vi "split by cursor pos.vi"(8 "error in":errorcluster, 11 "input":string) -> (0 "error out":errorcluster, 1 "Last cursor pos":cluster{i32, i32}, 2 "Sections":string[](array[string]), 3 "data":cluster{"Y":i32, "X":i32, "Text":string}[](array[cluster]))   [LabVIEW 2018]
uses:
  CAEN globals.vi
  <vilib>/regexp/Match Regular Expression.xnode
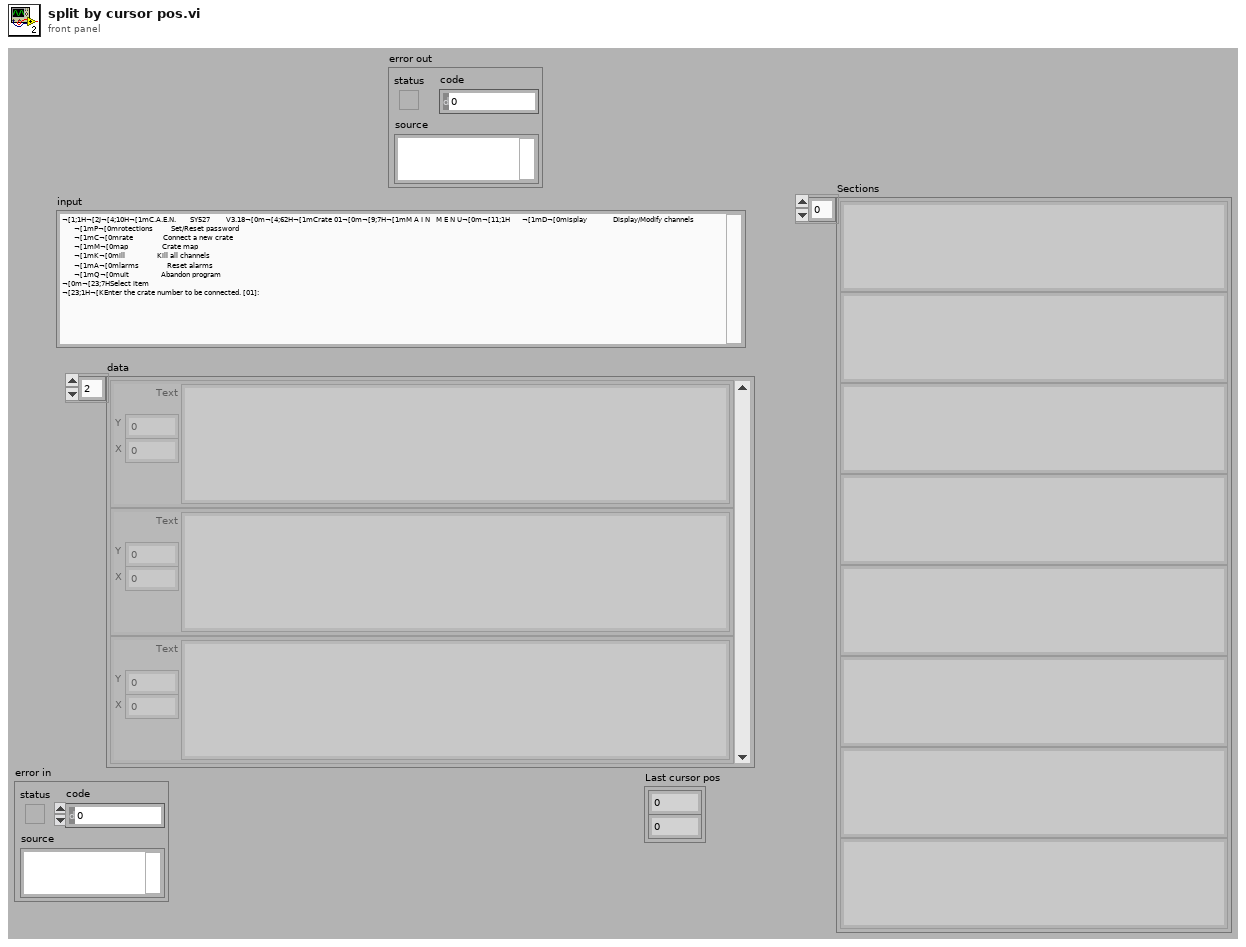
[diagram p1: front panel]
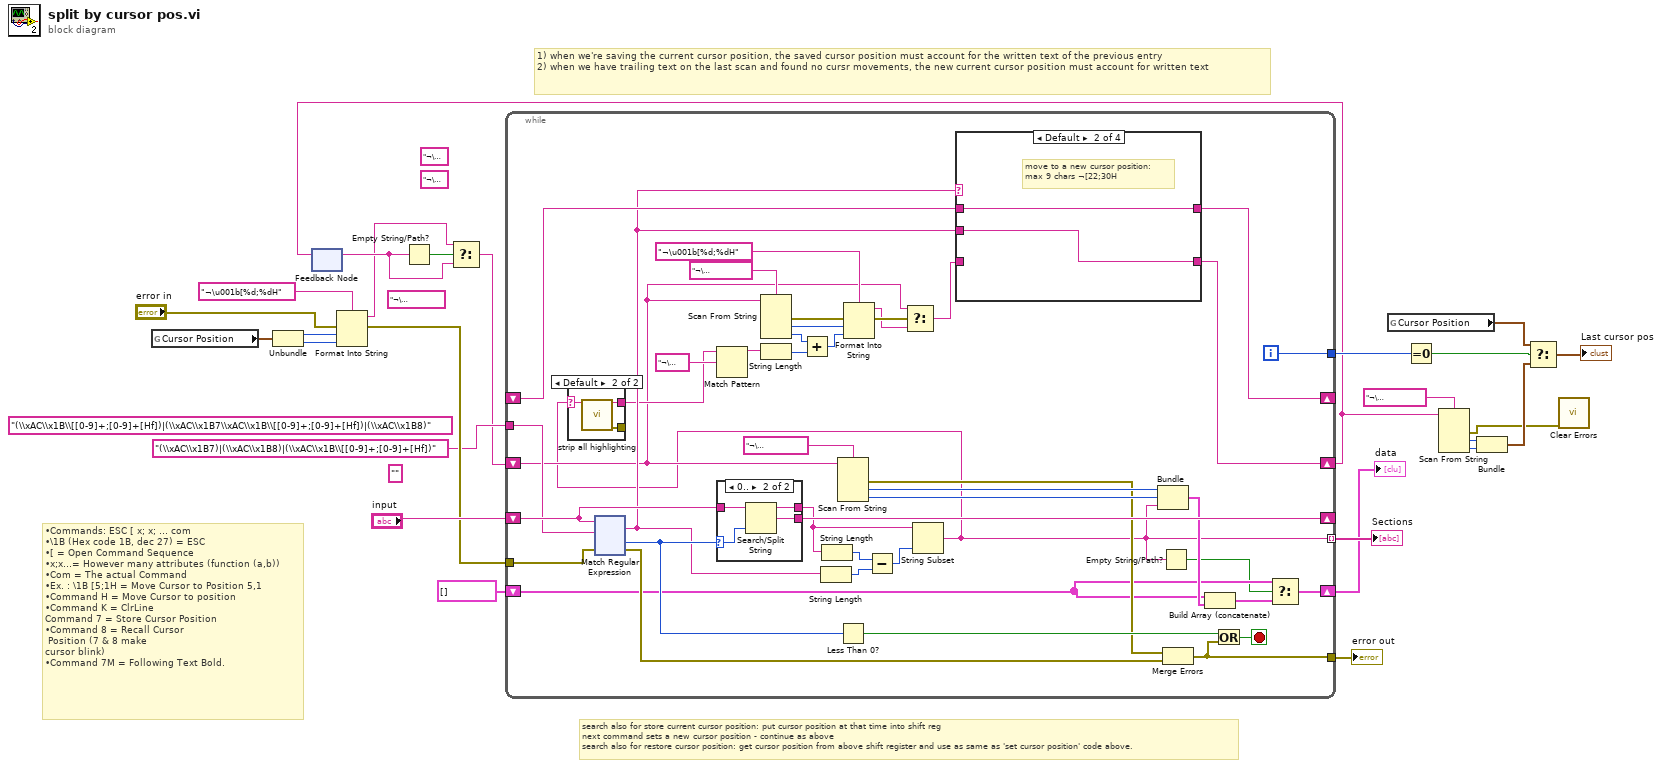
[diagram p0: block diagram]
diagram:
  (unwired) "¬\u001b8" ("s? t:f")
  (unwired) "¬\u001b7" ("s? t:f")
  (unwired) "¬\u001b[21;0H" ("s? t:f")
  (unwired) "(\\xAC\\x1B\\[[0-9]+;[0-9]+[Hf])|(\\xAC\\x1B7\\xAC\\x1B\\[[0-9]+;[0-9]+[Hf])|(\\xAC\\x1B8)" ("search string")
  (unwired) "" ("whole match")
  # "1) when we're saving the current cursor position, the saved cursor position must account for the written text of the previous entry\n2) when we have trailing text on the last scan and found no cursr movements, the new current cursor position must account for written text"
  # "•Commands: ESC [ x; x; … com \n•\\1B (Hex code 1B, dec 27) = ESC \n•[ = Open Command Sequence \n•x;x…= However many attributes (function (a,b)) \n•Com = The actual Command \n•Ex. : \\1B [5;1H = Move Cursor to Position 5,1 \n•Command H = Move Cursor to position \n•Command K = ClrLine\nCommand 7 = Store Cursor Position \n•Command 8 = Recall Cursor\n Position (7 & 8 make \ncursor blink) \n•Command 7M = Following Text Bold."
  # "search also for store current cursor position: put cursor position at that time into shift reg\nnext command sets a new cursor position - continue as above\nsearch also for restore cursor position: get cursor position from above shift register and use as same as 'set cursor position' code above."
  n1 = global read "CAEN globals.vi" "Cursor Position"() -> (w3:cluster{i32, i32})
  n2 = Unbundle(w3) -> (w21:i32, w22:i32)
  n3 = feedback #1() -> (w16:string)  [unwired: 1 in]
  n4 = Format Into String(format string="¬\u001b[%d;%dH" ("search string"), error in="error in", w21, w22) -> (resulting string=w15:string, error out=w18:errorcluster)  [unwired: 1 in]
  n5 = Empty String/Path?(string/path=w16) -> (empty?=w17:bool)
  n6 = Select(t=w15, s=w17, f=w16) -> (s? t:f=w1:string)
  n7 = while {
    shift-right: [w67] -> _
    shift-left: "input" -> [w68]
    tunnel: [w28] -> w24 mode=indexing
    shift-right: [w43] -> w2
    shift-left: w1 -> [w29]
    tunnel: [w51] -> w23
    tunnel: w18 -> [w64]
    tunnel: "(\\xAC\\x1B7)|(\\xAC\\x1B8)|(\\xAC\\x1B\\[[0-9]+;[0-9]+[Hf])" ("search string") -> [w63]
    shift-right: [w52] -> _
    shift-left: _ -> [w53]
    shift-right: [w47] -> w13
    shift-left: cluster{i32, i32, "result string":string}[] [] -> [w46]
    tunnel: [w44] -> w10
    i -> [w44]
    stop <- w65 stop-if-true
    n8 = xnode "Match Regular Expression"("input string"=w68, "regular expression"=w63, "error in"=w64) -> ("whole match"=w42:string, "offset past match"=w66:i32, "error out"=w62:errorcluster)  [unwired: 3 in, 2 out]
    n9 = case shown="0.." w66 {
      selector: w66 -> [_ w82]
      tunnel: w68 -> [w79 w83]
      tunnel: [w79 w80] -> w57
      tunnel: [_ w81] -> w67
      frame Default {
      }
      frame 0.. {
        n10 = Search/Split String(string=w83, offset (0)=w82) -> (substring before match=w80:string, match + rest of string=w81:string)  [unwired: 1 in, 1 out]
      }
    }
    n11 = Scan From String(format string="¬\u001b[%d;%d" ("search string"), input string=w29) -> (error out=w35:errorcluster, output 1=w32:i32, output 2=w31:i32)  [unwired: 4 in, 2 out]
    n12 = String Length(string=w42) -> (length=w59:i32)
    n13 = String Length(string=w57) -> (length=w60:i32)
    n14 = Scan From String(format string="¬\u001b[%d;%d" ("search string"), input string=w29) -> (error out=w50:errorcluster, output 1=w55:i32, output 2=w54:i32)  [unwired: 4 in, 2 out]
    n15 = Less Than 0?(x=w66) -> (x < 0?=w61:bool)
    n16 = Subtract(x=w60, y=w59) -> (x-y=w58:i32)
    n17 = String Subset(string=w57, length (rest)=w58) -> (substring=w28:string)  [unwired: 1 in]
    n18 = case shown="Default" w28 {
      selector: w28 -> [w69 w71]
      tunnel: [w69 w72] -> w40
      tunnel: [_ w70] -> _
      frame "" {
      }
      frame Default {
        n19 = call "strip all highlighting.vi"("input string"=w71) -> ("stripped output"=w72:string, "error out"=w70:errorcluster)  [unwired: 9 in, 4 out]
      }
    }
    n20 = Match Pattern(string=w40, regular expression="¬\u001b\\[." ("clear line")) -> (before substring=w39:string)  [unwired: 1 in, 3 out]
    n21 = String Length(string=w39) -> (length=w36:i32)
    n22 = Add(x=w31, y=w36) -> (x+y=w30:i32)
    n23 = Format Into String(format string="¬\u001b[%d;%dH" ("search string"), error in=w35, w32, w30) -> (resulting string=w33:string, error out=w34:errorcluster)  [unwired: 1 in]
    n24 = Select(t=w29, s=w34, f=w33) -> (s? t:f=w27:string)
    n25 = case shown="Default" w42 {
      tunnel: [w73 w74 w76 w78] -> w43
      tunnel: w42 -> [_ w74 _ _]
      tunnel: [w73 w75 w77 w78] -> w52
      tunnel: w53 -> [w73 w75 w77 _]
      tunnel: w27 -> [_ _ w76 w78]
      frame "¬\u001b8" {
        # "restore the stored cusror position"
      }
      frame Default {
        # "move to a new cursor position:\nmax 9 chars ¬[22;30H"
      }
      frame "" {
        # "No input: propagate"
      }
      frame "¬\u001b7" {
        # "store current cursor positon\n and move to \na new one: minimum 10 chars ¬7¬[5;1H"
      }
    }
    n26 = Bundle(w55, w54, "input"=w28) -> (w49:cluster{i32, i32, "input":string})  [unwired: 1 in]
    n27 = Empty String/Path?(string/path=w28) -> (empty?=w45:bool)
    n28 = Merge Errors(w50, w62) -> (w51:errorcluster)
    n29 = Build Array (concatenate)(w46, w49) -> (w48:cluster{i32, i32, "input":string}[])
    n30 = Or(x=w61, y=w51) -> (x .or. y?=w65:bool)
    n31 = Select(t=w46, s=w45, f=w48) -> (s? t:f=w47:cluster{i32, i32, "input":string}[])
  }
  "Sections" <- w24
  "error out" <- w23
  "data" <- w13
  n32 = feedback-in #1(w2) -> ()
  n33 = global read "CAEN globals.vi" "Cursor Position"() -> (w12:cluster{i32, i32})
  n34 = Equal To 0?(x=w10) -> (x = 0?=w9:bool)
  n35 = Scan From String(format string="¬\u001b[%d;%d" ("search string"), input string=w2) -> (error out=w4:errorcluster, output 1=w8:i32, output 2=w5:i32)  [unwired: 4 in, 2 out]
  n36 = Bundle(w8, w5) -> (w6:cluster{i32, i32})  [unwired: 1 in]
  n37 = Select(t=w12, s=w9, f=w6) -> (s? t:f=→"Last cursor pos":cluster{i32, i32})
  n38 = call <vilib>:"Clear Errors.vi"("error in (no error)"=w4) -> ()  [unwired: 5 in, 2 out]
